vi "LuaVIEW Info_srv.vi"(7 "certificate":string) -> (8 "info":string, 15 "error out":errorcluster)   [LabVIEW 2012]
uses:
  clientsrv/typedefs/t_ClientSrv Access Levels.ctl
  typedefs/et_LuaVIEW CIN Actions.ctl
  typedefs/t_LuaVIEW CIN Spinlocked Actions.ctl
  glb_LuaVIEW Configuration Globals.vi
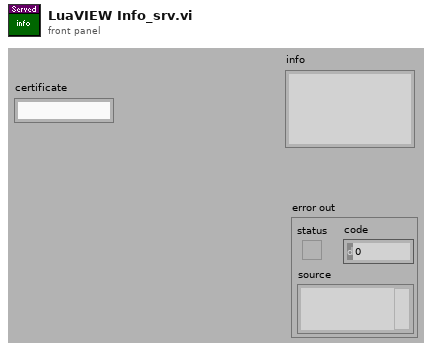
[diagram p1: front panel]
types:
  T1 = typedef "t_ClientSrv Access Levels.ctl" = enum16{"observer", "operator", "local"}
  T2 = typedef "et_LuaVIEW CIN Actions.ctl" = enum16{"checksynopsis", "_open", "_registerpublic", "_registerexport", "__never_an_error_result_ns", "luaversion", "cinversion", "_totals", "_taskcount", "pathological", "_unregnextpublic", "registryusecount", "__per_state_actions", "regsetprivate", "regsetindex", "regsetmodule", "_revokeexports", "_usepublic", "prepare", "compile", "execute", "call", "unregstaterefs", "_close", "pullboolean", "pullnumber", "pullI8", "pullU8", "pullI16", "pullU16", "pullI32", "pullU32", "pullobject", "pullrefnum", "pullstring", "pullflat", "pushflat", "pushobject", "getattribute", "setattribute", "stacktostring", "_startyieldtest", "_endyieldtest", "_pollprintbuffer", "__never_an_error_result_ps", "_pollexport", "setclone", "forcecleanup", "gettop", "clearstack", "insert", "pushboolean", "pushnumber", "pushrefnum", "pushstring", "pushnil", "pushvalue", "gettaskref", "settaskref"}
  T3 = typedef "t_LuaVIEW CIN Spinlocked Actions.ctl" = enum16{"totals", "taskcount", "open", "registerpublic", "registerexport", "revokeexports", "unregnextpublic", "usepublic", "pollexport", "close", "startyieldtest", "endyieldtest", "pollprintbuffer"}
  T4 = enum32{"invalid app kind", "Development System", "Run Time System", "Student Edition", "Embedded LabVIEW", "Evaluation", "Custom"}
  T5 = cluster{"totalFreeSize":i64, "maxFreeSize":i64, "nFreeblocks":i64, "totAllocSize":i64, "maxAllocSize":i64, "nPointers":i64, "nUnlockedHdls":i64, "nLockedHdls":i64, "reserved1":i32, "reserved2":i32, "reserved3":i32, "reserved4":i32}
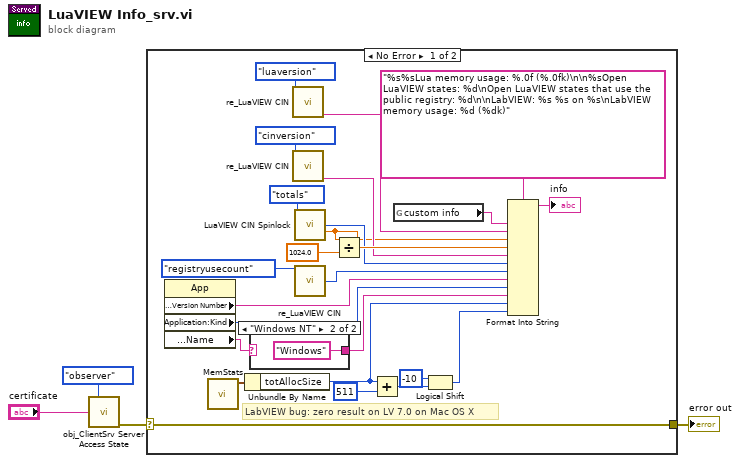
[diagram p0: block diagram]
diagram:
  n1 = call "obj_ClientSrv Server Access State.vi"("access level"=t_ClientSrv_Access_Levels."observer", "certificate in"="certificate") -> ("error out"=w1:errorcluster)  [unwired: 11 in, 2 out]
  n2 = case shown="No Error" w1 {
    selector: w1 -> [w29 w32]
    tunnel: [w29 w32] -> w2
    frame No Error {
      # "LabVIEW bug: zero result on LV 7.0 on Mac OS X"
      n3 = property class="App"() -> ("Application:Version Number"=w14:string, "Application:Kind"=w13:T4, "Operating System:Name"=w12:string)  [unwired: 2 in, 2 out]
      n4 = call <vilib>:"MemStats.vi"() -> ("AZ memStats"=w28:T5)  [unwired: 5 in, 2 out]
      n5 = Unbundle By Name(w28) -> ("totAllocSize"=w15:i64)
      n6 = case shown="\"Windows NT\"" w12 {
        selector: w12 -> [w30 _]
        tunnel: [w30 "Windows"] -> w11
        frame Default {
        }
        frame "Windows NT" {
        }
      }
      n7 = call "re_LuaVIEW CIN.vi"("action"=et_LuaVIEW_CIN_Actions."luaversion") -> ("string out"=w9:string)  [unwired: 8 in, 6 out]
      n8 = call "re_LuaVIEW CIN.vi"("action"=et_LuaVIEW_CIN_Actions."cinversion") -> ("string out"=w17:string)  [unwired: 8 in, 6 out]
      n9 = call "LuaVIEW CIN Spinlock.vi"("action"=t_LuaVIEW_CIN_Spinlocked_Actions."totals") -> ("index out"=w16:i32, "number out"=w10:dbl)  [unwired: 8 in, 5 out]
      n10 = call "re_LuaVIEW CIN.vi"("action"=et_LuaVIEW_CIN_Actions."registryusecount") -> ("index out"=w6:i32)  [unwired: 8 in, 6 out]
      n11 = Divide(x=w10, y=1024.0) -> (x/y=w18:dbl)
      n12 = Add(x=w15, y=511) -> (x+y=w21:i64)
      n13 = global read "glb_LuaVIEW Configuration Globals.vi" "custom info"() -> (w8:string)
      n14 = Logical Shift(y=-10, x=w21) -> (x << y=w19:i64)
      n15 = Format Into String(format string="%s%sLua memory usage: %.0f (%.0fk)\n\n%sOpen LuaVIEW states: %d\nOpen LuaVIEW states that use the public registry: %d\n\nLabVIEW: %s %s on %s\nLabVIEW memory usage: %d (%dk)", w8, w9, w10, w18, w17, w16, w6, w14, w13, w11, w15, w19) -> (resulting string=→"info":string)  [unwired: 2 in, 1 out]
    }
    frame Error {
    }
  }
  "error out" <- w2
